vi "Parse Scaling Constant Table.vi"(7 "Scaling Constant Table":string, 8 "error in (no error)":errorcluster, 11 "Variant in":variant) -> (0 "error out":errorcluster, 3 "Variant out":variant)   [LabVIEW 2021]
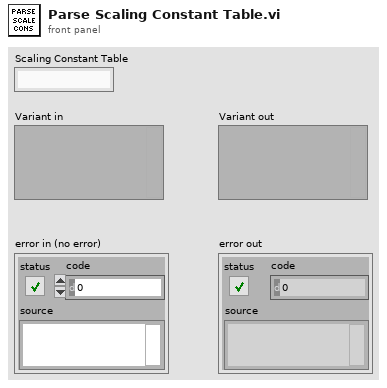
[diagram p1: front panel]
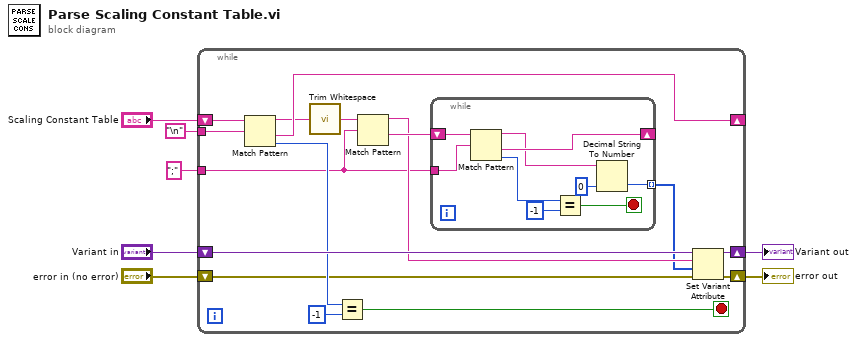
[diagram p0: block diagram]
diagram:
  n1 = while {
    shift-right: [w23] -> w5
    shift-left: "Variant in" -> [w22]
    shift-right: [w17] -> _
    shift-left: "Scaling Constant Table" -> [w21]
    tunnel: ";" -> [w12]
    tunnel: "\n" -> [w11]
    shift-right: [w9] -> w1
    shift-left: "error in (no error)" -> [w10]
    stop <- w18 stop-if-true
    n2 = Match Pattern(string=w21, regular expression=w11) -> (before substring=w16:string, after substring=w17:string, offset past match=w20:i32)  [unwired: 1 in, 1 out]
    n3 = call <vilib>:"Trim Whitespace.vi"("string"=w16) -> ("trimmed string"=w8:string)  [unwired: 1 in]
    n4 = Equal?(x=w20, y=-1) -> (x = y?=w18:bool)
    n5 = Match Pattern(string=w8, regular expression=w12) -> (before substring=w14:string, after substring=w15:string)  [unwired: 1 in, 2 out]
    n6 = while {
      shift-right: [w31] -> _
      shift-left: w15 -> [w32]
      tunnel: w12 -> [w27]
      tunnel: [w24] -> w13 mode=indexing
      stop <- w28 stop-if-true
      n7 = Match Pattern(string=w32, regular expression=w27) -> (before substring=w25:string, after substring=w31:string, offset past match=w29:i32)  [unwired: 1 in, 1 out]
      n8 = Equal?(x=w29, y=-1) -> (x = y?=w28:bool)
      n9 = Decimal String To Number(string=w25, default (0L)=u32 0 ("default (0 I32)")) -> (number=w24:u32)  [unwired: 1 in, 1 out]
    }
    n10 = Set Variant Attribute(Variant=w22, name=w14, value=w13, error in=w10) -> (Variant out=w23:variant, error out=w9:errorcluster)  [unwired: 1 out]
  }
  "Variant out" <- w5
  "error out" <- w1
